vi "MSSQL_SelectExecute.vi"(6 "异常输入":errorcluster, 7 "是否有数据输出":bool, 8 "执行语句":string, 9 "connection reference":T1) -> (0 "异常输出":errorcluster, 1 "变体转换后数据":string[][](array[string]), 2 "操作结果":bool, 3 "connection reference 2":T1, 4 "完整数据":variant[][](array[variant]))   [LabVIEW 2018]
uses:
  <vilib>/addons/database/Connection.llb/Conn ObjectReference.ctl
  <vilib>/addons/database/Connection.llb/Conn Execute.vi
  <vilib>/addons/database/Recordset.llb/Rec Fetch Recordset Data (R).vi
  <vilib>/addons/database/Recordset.llb/Rec Destroy - Connection.vi
  <vilib>/addons/database/NI_Database_API.lvlib
panel:
  # "sql语句执行操作"
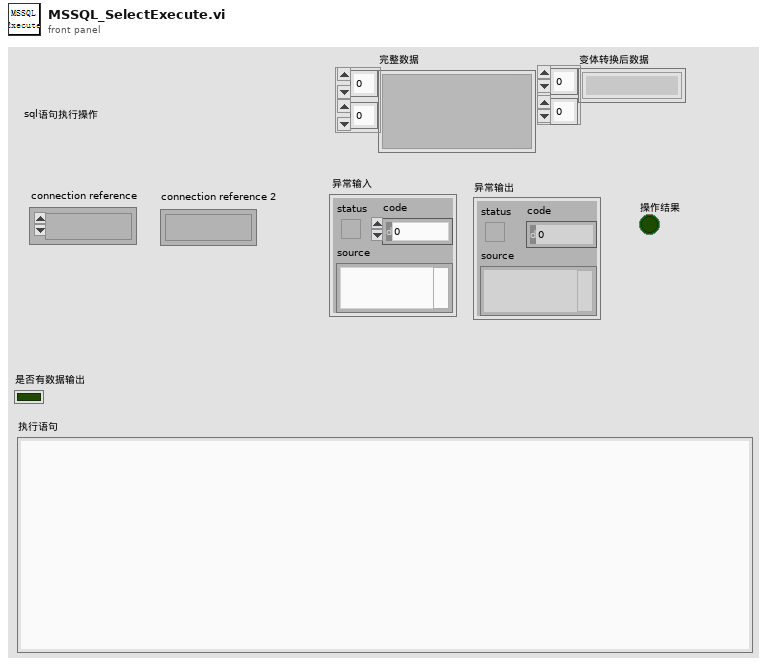
[diagram p1: front panel]
types:
  T1 = typedef "NI_Database_API.lvlib/Conn ObjectReference.ctl" = refnum<k1>
  T2 = typedef "NI_Database_API.lvlib/Rec ObjectReference.ctl" = refnum<k1>
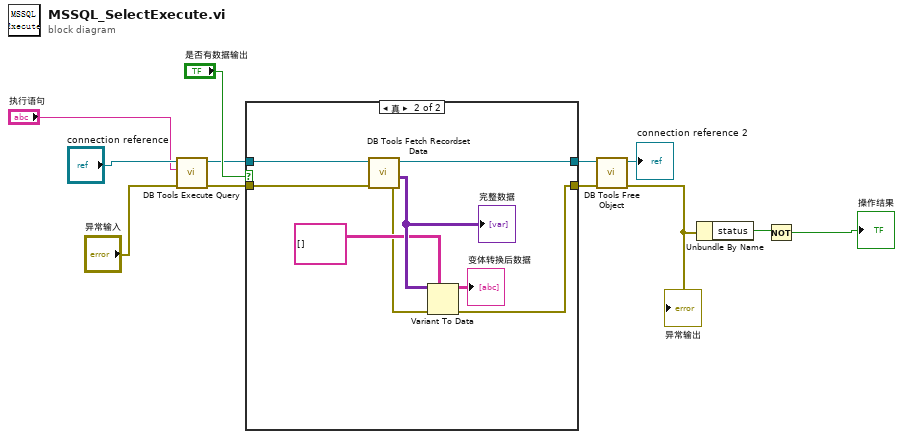
[diagram p0: block diagram]
diagram:
  n1 = call-poly <vilib>:"DB Tools Execute Query.vi"("error in (no error)"="异常输入", "SQL query"="执行语句", "connection reference"="connection reference") -> ("error out"=w3:errorcluster, "recordset reference"=w4:T2)  [unwired: 5 in]
  n2 = case shown="真" "是否有数据输出" {
    tunnel: w4 -> [w14 w22]
    tunnel: w3 -> [w13 w21]
    tunnel: [w14 w20] -> w2
    tunnel: [w13 w16] -> w1
    frame False {
    }
    frame True {
      n3 = call-poly <vilib>:"DB Tools Fetch Recordset Data.vi"("error in (no error)"=w21, "recordset reference"=w22) -> ("error out"=w17:errorcluster, "recordset data"=w19:variant[][], "recordset reference out"=w20:T2)  [unwired: 3 in]
      "完整数据" <- w19
      n4 = Variant To Data(error in=w17, type=string[][] [], Variant=w19) -> (data=→"变体转换后数据":string[][], error out=w16:errorcluster)
    }
  }
  n5 = call-poly <vilib>:"DB Tools Free Object.vi"("error in (no error)"=w1, "recordset reference"=w2) -> ("error out"=w9:errorcluster, "connection reference"=→"connection reference 2":T1)  [unwired: 8 in]
  "异常输出" <- w9
  n6 = Unbundle By Name(w9) -> ("status"=w8:bool)
  n7 = Not(x=w8) -> (.not. x?=→"操作结果":bool)
